vi "saveToFits.vi"(6 "hwInfo":string="Initial Time", 7 "errorList":string="Initial Time", 8 "error in (no error)":errorcluster, 9 "time":dbl[](array[numeric]), 10 "value":dbl[](array[numeric]), 11 "ElectrometerController in":refnum<class "ElectrometerController.lvclass">) -> (0 "error out":errorcluster, 1 "fileSize":i64, 2 "Path":path, 3 "ElectrometerController out":refnum<class "ElectrometerController.lvclass">)   [LabVIEW 2016, in "ElectrometerController.lvclass"]
uses:
  ElectrometerController.lvclass
  cfitsio/cftsio.lvclass
  ElectrometerController.lvclass/ElectrometerController.ctl
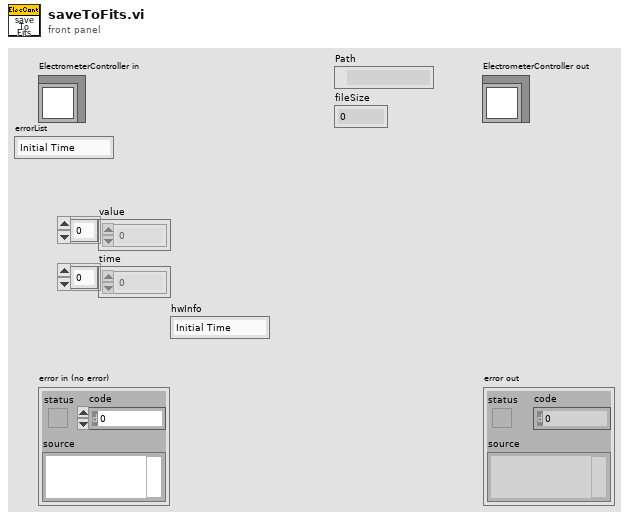
[diagram p1: front panel]
types:
  T1 = typedef "ElectrometerTypedefs.lvlib/Reading.ctl" = cluster{"intensity":dbl, "Unit":string, "temperature":dbl}
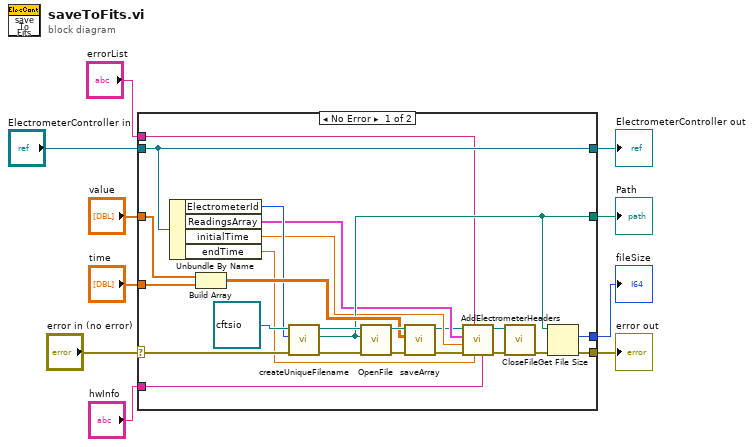
[diagram p0: block diagram]
diagram:
  n1 = case shown="No Error" "error in (no error)" {
    selector: "error in (no error)" -> [w26 w35]
    tunnel: [w21 w36] -> w8
    tunnel: "ElectrometerController in" -> [w21 w36]
    tunnel: "value" -> [w30 _]
    tunnel: "time" -> [w29 _]
    tunnel: [w25 _] -> w5
    tunnel: [w24 _] -> w4
    tunnel: [w22 w35] -> w3
    tunnel: "errorList" -> [w12 _]
    tunnel: "hwInfo" -> [w11 _]
    frame No Error {
      n2 = Unbundle By Name(w21) -> ("ElectrometerId"=w20:enum16{"", "ID1", "ID2"}, "ReadingsArray"=w14:T1[], "initialTime"=w15:dbl, "endTime"=w16:dbl)
      n3 = Build Array(w30, w29) -> (w28:dbl[][])
      n4 = call "createUniqueFilename.vi"("error in (no error)"=w26, "ElectrometerId"=w20, "cftsio in"=refnum<class "cftsio.lvclass"> refnum ("cftsio.lvclass")) -> ("error out"=w32:errorcluster, "Path"=w25:path, "cftsio out"=w33:refnum<class "cftsio.lvclass">)  [unwired: 6 in]
      n5 = call "OpenFile.vi"("error in (no error)"=w32, "Path"=w25, "cftsio in"=w33) -> ("error out"=w27:errorcluster, "cftsio out"=w31:refnum<class "cftsio.lvclass">)  [unwired: 7 in]
      n6 = call "saveArray.vi"("error in (no error)"=w27, "Array"=w28, "cftsio in"=w31) -> ("error out"=w19:errorcluster, "cftsio out"=w13:refnum<class "cftsio.lvclass">)  [unwired: 7 in]
      n7 = call "AddElectrometerHeaders.vi"("hwInfo"=w11, "endTime"=w16, "errorList"=w12, "error in (no error)"=w19, "initialTime"=w15, "ReadingsArray"=w14, "cftsio in"=w13) -> ("error out"=w18:errorcluster, "cftsio out"=w17:refnum<class "cftsio.lvclass">)  [unwired: 3 in]
      n8 = call "CloseFile.vi"("error in (no error)"=w18, "cftsio in"=w17) -> ("error out"=w23:errorcluster)  [unwired: 8 in, 1 out]
      n9 = Get File Size(file=w25, error in=w23) -> (size (in bytes)=w24:i64, 0:w22:errorcluster)  [unwired: 1 out]
    }
    frame Error {
    }
  }
  "error out" <- w3
  "ElectrometerController out" <- w8
  "Path" <- w5
  "fileSize" <- w4
